vi "Send Configure Trigger Source [TRG].vi"(7 "Message Priority (Normal)":T1=enum."Normal", 8 "error in (no error)":errorcluster, 9 "source (Immediate)":i32(ring) items=["Immediate", "External", "Software", "TTL0", "TTL1", "TTL2", "TTL3", "TTL4", "TTL5", "TTL6", "TTL7", "ECL0", "ECL1", "PXI Star", "RTSI 0", "RTSI 1", "RTSI 2", "RTSI 3", "RTSI 4", "RTSI 5", "RTSI 6"], 10 "channel name (\"CHANNEL1\")":string="CHANNEL1", 11 "Message Enqueuer":refnum<class "Message Enqueuer.lvclass">) -> (0 "error out":errorcluster, 3 "Message Enqueuer out":refnum<class "Message Enqueuer.lvclass">)   [LabVIEW 2015, in "CS++DCPwr.lvlib" / "Configure Trigger Source [TRG] Msg.lvclass"]
doc: "Sends the <B>CS++DCPwr.lvlib:Configure Trigger Source [TRG] Msg.lvclass</B> message.\n\n<B>CS++DCPwr.lvlib:CS++DCPwr.lvclass:Configure Trigger Source [TRG].vi</B> Description:\n\nThis VI configures the trigger source to which the power supply responds after you call IviDCPwr Initiate [TRG]. When the power supply receives a trigger signal on the source you specify, it changes its current and voltage outputs.\n\nYou configure the triggered current and voltage outputs with the\nIviDCPwr Configure Triggered Current Limit [TRG] and \nIviDCPwr Configure Triggered Voltage Level [TRG] VIs. \n\nNotes:\n\n(1) This VI is part of the IviDCPwrTrigger [TRG] extension group."
uses:
  Configure Trigger Source [TRG] Msg.lvclass
  <vilib>/ActorFramework/Message Enqueuer/Message Enqueuer.lvclass
  <vilib>/ActorFramework/Message Enqueuer/Message Priority.ctl
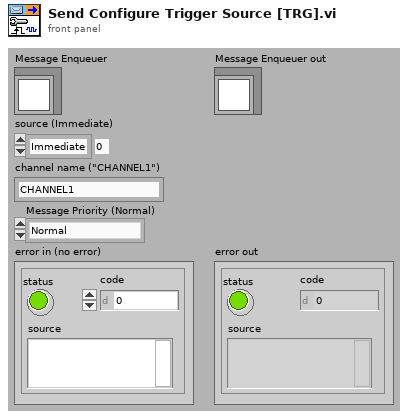
[diagram p1: front panel]
types:
  T1 = typedef "Actor Framework.lvlib/Message Enqueuer.lvclass/Message Priority.ctl" = enum16{"Low", "Normal", "High"}
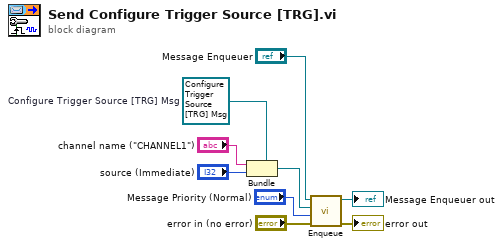
[diagram p0: block diagram]
diagram:
  w3 = refnum<class "Configure Trigger Source [TRG] Msg.lvclass"> refnum  # Configure Trigger Source [TRG] Msg
  n1 = Bundle(cluster=w3, "channel name (\"CHANNEL1\")", "source (Immediate)") -> (w6:refnum<class "Configure Trigger Source [TRG] Msg.lvclass">)
  n2 = call <vilib>:"Enqueue.vi"("error in (no error)"="error in (no error)", "Message Priority (Normal)"="Message Priority (Normal)", "Message"=w6, "Message Enqueuer in"="Message Enqueuer") -> ("error out"=→"error out":errorcluster, "Message Enqueuer out"=→"Message Enqueuer out":refnum<class "Message Enqueuer.lvclass">)  [unwired: 6 in]
